vi "Create Published Group.vi"(11 "Group":refnum<class "Group.lvclass">) -> (3 "Published Group":T1 {"Publish Port" format="%.0x"; "Publish Address" format="%<%H:%M:%S%3u>T"; "Last Publish" format="%<%H:%M:%S%3u>T"})   [LabVIEW 2020, in "Vecto.lvlib" / "RemoteDataService.lvclass"]
uses:
  RemoteDataService.lvclass
  Group/Group.lvclass
  Published Group.ctl
  Group/Group.lvclass/Group.ctl
  RemoteDataService.lvclass/RemoteDataService.ctl
  Group Config/Group Config.lvclass
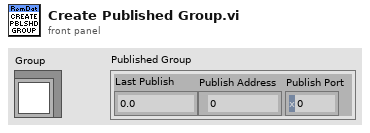
[diagram p1: front panel]
types:
  T1 = typedef "Vecto.lvlib/RemoteDataService.lvclass/Published Group.ctl" = cluster{"Last Publish":dbl, "Publish Address":u32, "Publish Port":u16}
  T2 = typedef "VectoConfig.lvlib/Publish Config.ctl" = cluster{"Address":string, "Port":u16}
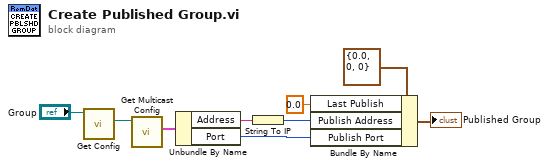
[diagram p0: block diagram]
diagram:
  n1 = call "Get Config.vi"("Group in"="Group") -> ("Config"=w6:refnum<class "Group Config.lvclass">)  [unwired: 8 in, 2 out]
  n2 = call "Get Multicast Config.vi"("Group Config in"=w6) -> ("Multicast Config"=w4:T2)  [unwired: 8 in, 2 out]
  n3 = Unbundle By Name(w4) -> ("Address"=w3:string, "Port"=w1:u16)
  n4 = String To IP(1:w3) -> (0:w2:u32)
  n5 = Bundle By Name(cluster=T1 {"Last Publish"=0.0, "Publish Address"=0, "Publish Port"=0} ("Published Group"), "Last Publish"=0.0, "Publish Address"=w2, "Publish Port"=w1) -> (→"Published Group":T1)
